vi "DriveForDistanceController.vi"(0 "Distance":dbl=300.0, 5 "Angle":dbl=164.32, 9 "SensorData":T3={"LeftDistance"=261.910213470459, "RightDistance"=383.47772216796875, "LeftVelocity"=63.071308056640625, "RightVelocity"=41.74135772460938, "Angle"=164.32, "Location"={-465.44436408260333, -5.658206958861253}}, 11 "Gains":T2={"FFV"=0.0097, "FFA"=0.002, "Vel PID"={"P"=0.0, "I"=0.0, "D"=0.0}}, 12 "Trackwidth":dbl=25.0 format="%#_13g", 13 "Reset":bool) -> (4 "Left Speed":dbl, 6 "Right Speed":dbl=-2.7755575615628914e-17, 10 "Done":bool=TRUE, 14 "Graph":cluster{cluster{"x":dbl, "y":dbl}[]}[](graph)=[{[{"x"=-182.84036380917772, "y"=-102.60157058324037}, {"x"=-188.50213040089133, "y"=-100.61551946079776}, {"x"=-194.16389699260495, "y"=-98.62946833835514}, {"x"=-199.82566358431856, "y"=-96.64341721591252}, {"x"=-205.48743017603218, "y"=-94.65736609346989}, {"x"=-211.1491967677458, "y"=-92.67131497102727}, {"x"=-216.8109633594594, "y"=-90.68526384858465}, {"x"=-222.47272995117302, "y"=-88.69921272614204}, {"x"=-228.13449654288664, "y"=-86.71316160369942}, {"x"=-233.79626313460025, "y"=-84.7271104812568}, {"x"=-239.45802972631387, "y"=-82.74105935881417}, {"x"=-245.11979631802748, "y"=-80.75500823637157}, {"x"=-250.7815629097411, "y"=-78.76895711392893}, {"x"=-256.44332950145474, "y"=-76.78290599148632}, {"x"=-262.1050960931683, "y"=-74.7968548690437}, {"x"=-267.76686268488197, "y"=-72.81080374660108}, {"x"=-273.42862927659553, "y"=-70.82475262415846}, {"x"=-279.0903958683092, "y"=-68.83870150171583}, {"x"=-284.75216246002276, "y"=-66.85265037927323}, {"x"=-290.41392905173643, "y"=-64.8665992568306}, {"x"=-296.07569564345, "y"=-62.88054813438798}, {"x"=-301.73746223516366, "y"=-60.89449701194536}, {"x"=-307.3992288268772, "y"=-58.908445889502744}, {"x"=-313.0609954185909, "y"=-56.922394767060126}, {"x"=-318.72276201030445, "y"=-54.9363436446175}, {"x"=-324.3845286020181, "y"=-52.950292522174884}, {"x"=-330.0462951937317, "y"=-50.964241399732266}, {"x"=-335.70806178544535, "y"=-48.97819027728964}, {"x"=-341.3698283771589, "y"=-46.992139154847024}, {"x"=-347.0315949688726, "y"=-45.006088032404406}, {"x"=-352.69336156058614, "y"=-43.02003690996179}, {"x"=-358.3551281522998, "y"=-41.033985787519164}, {"x"=-364.01689474401337, "y"=-39.047934665076546}, {"x"=-369.67866133572704, "y"=-37.06188354263392}, {"x"=-375.3404279274406, "y"=-35.075832420191304}, {"x"=-381.0021945191543, "y"=-33.08978129774869}, {"x"=-386.66396111086783, "y"=-31.10373017530607}, {"x"=-392.3257277025815, "y"=-29.11767905286345}, {"x"=-397.98749429429506, "y"=-27.131627930420834}, {"x"=-403.64926088600873, "y"=-25.145576807978216}, {"x"=-409.3110274777223, "y"=-23.159525685535584}, {"x"=-414.97279406943596, "y"=-21.173474563092967}, {"x"=-420.6345606611495, "y"=-19.18742344065035}, {"x"=-426.2963272528632, "y"=-17.20137231820773}, {"x"=-431.95809384457675, "y"=-15.215321195765114}, {"x"=-437.6198604362904, "y"=-13.229270073322496}, {"x"=-443.281627028004, "y"=-11.243218950879879}, {"x"=-448.94339361971765, "y"=-9.257167828437247}, {"x"=-454.6051602114312, "y"=-7.271116705994629}, {"x"=-460.2669268031449, "y"=-5.2850655835520115}, {"x"=-461.21055456843044, "y"=-4.954057063144916}, {"x"=-465.92869339485844, "y"=-3.299014461109394}]}, {[{"x"=-465.44436408260333, "y"=-5.658206958861253}, {"x"=-476.9977978243892, "y"=-2.415034318657715}]}, {[{"x"=-463.7557202118273, "y"=-4.061256379649985}]}, {[{"x"=-440.44436408260333, "y"=-5.658206958861253}, {"x"=-440.9906740642582, "y"=-0.46041468841727085}, {"x"=-442.6057276415383, "y"=4.51020911803375}, {"x"=-445.21893922322965, "y"=9.036424348450575}, {"x"=-448.7160989236319, "y"=12.9204136780736}, {"x"=-452.94436408260333, "y"=15.992428135749712}, {"x"=-457.71893922322965, "y"=18.118205948517584}, {"x"=-462.83115250091197, "y"=19.20484042534558}, {"x"=-468.0575756642947, "y"=19.20484042534558}, {"x"=-473.169788941977, "y"=18.118205948517588}, {"x"=-477.94436408260333, "y"=15.992428135749716}, {"x"=-482.1726292415748, "y"=12.920413678073608}, {"x"=-485.669788941977, "y"=9.036424348450577}, {"x"=-488.28300052366836, "y"=4.510209118033757}, {"x"=-489.89805410094846, "y"=-0.4604146884172602}, {"x"=-490.44436408260333, "y"=-5.658206958861251}, {"x"=-489.89805410094846, "y"=-10.85599922930523}, {"x"=-488.28300052366836, "y"=-15.82662303575625}, {"x"=-485.669788941977, "y"=-20.35283826617308}, {"x"=-482.1726292415748, "y"=-24.236827595796104}, {"x"=-477.94436408260333, "y"=-27.308842053472212}, {"x"=-473.169788941977, "y"=-29.43461986624009}, {"x"=-468.0575756642947, "y"=-30.521254343068087}, {"x"=-462.831152500912, "y"=-30.521254343068087}, {"x"=-457.71893922322965, "y"=-29.434619866240094}, {"x"=-452.94436408260333, "y"=-27.30884205347223}, {"x"=-448.7160989236319, "y"=-24.236827595796118}, {"x"=-445.21893922322965, "y"=-20.352838266173087}, {"x"=-442.6057276415383, "y"=-15.826623035756276}, {"x"=-440.9906740642582, "y"=-10.855999229305251}, {"x"=-440.44436408260333, "y"=-5.65820695886126}]}, {[{"x"=-266.3585601807637, "y"=145.23719379541097}, {"x"=-269.7834396945887, "y"=177.82274570174297}, {"x"=-279.90839456691435, "y"=208.98415262694203}, {"x"=-296.29091568489616, "y"=237.35951155935658}, {"x"=-318.21500826362, "y"=261.70868315356114}, {"x"=-344.72248425392746, "y"=280.96749177060053}, {"x"=-374.65483975805995, "y"=294.29423505989314}, {"x"=-406.7038872091095, "y"=301.10647039088764}, {"x"=-439.46892944507306, "y"=301.1064703908877}, {"x"=-471.5179768961226, "y"=294.2942350598932}, {"x"=-501.4503324002551, "y"=280.96749177060053}, {"x"=-527.9578083905625, "y"=261.7086831535612}, {"x"=-549.8819009692864, "y"=237.35951155935658}, {"x"=-566.2644220872683, "y"=208.9841526269421}, {"x"=-576.3893769595938, "y"=177.82274570174303}, {"x"=-579.8142564734189, "y"=145.237193795411}, {"x"=-576.3893769595938, "y"=112.651641889079}, {"x"=-566.2644220872683, "y"=81.49023496387996}, {"x"=-549.8819009692864, "y"=53.114876031465386}, {"x"=-527.9578083905626, "y"=28.76570443726081}, {"x"=-501.4503324002552, "y"=9.506895820221445}, {"x"=-471.51797689612266, "y"=-3.8198474690712203}, {"x"=-439.46892944507323, "y"=-10.632082800065689}, {"x"=-406.7038872091096, "y"=-10.632082800065717}, {"x"=-374.65483975806, "y"=-3.8198474690712487}, {"x"=-344.7224842539276, "y"=9.506895820221331}, {"x"=-318.2150082636201, "y"=28.765704437260723}, {"x"=-296.29091568489616, "y"=53.11487603146533}, {"x"=-279.90839456691447, "y"=81.49023496387979}, {"x"=-269.7834396945887, "y"=112.65164188907889}, {"x"=-266.3585601807637, "y"=145.23719379541095}]}], 15 "Time Left":dbl=20.0)   [LabVIEW 2020]
uses:
  PurePursuit/RobotNeededPathData.ctl
panel:
  out "outputs":T1(graph)={"LeftValue"=0.0, "RightValue"=-2.7755575615628914e-17, 1.0, 0.5}
  out "Vel vs Target Vel":cluster{dbl, "TargetVel":dbl}(graph)={52.406332890625, "TargetVel"=52.70905958272918}
  in  "MaxDeAccel":dbl=120.0 format="%#_13g"
  in  "LookaheadDist":dbl=25.0
  in  "SlowSpeed":dbl=30.0 format="%#_13g"
  in  "SlowDistanceAtEnd":dbl=12.0 format="%#_13g"
  in  "MaxAccel":dbl=120.0
  in  "MaxVel":dbl=70.0
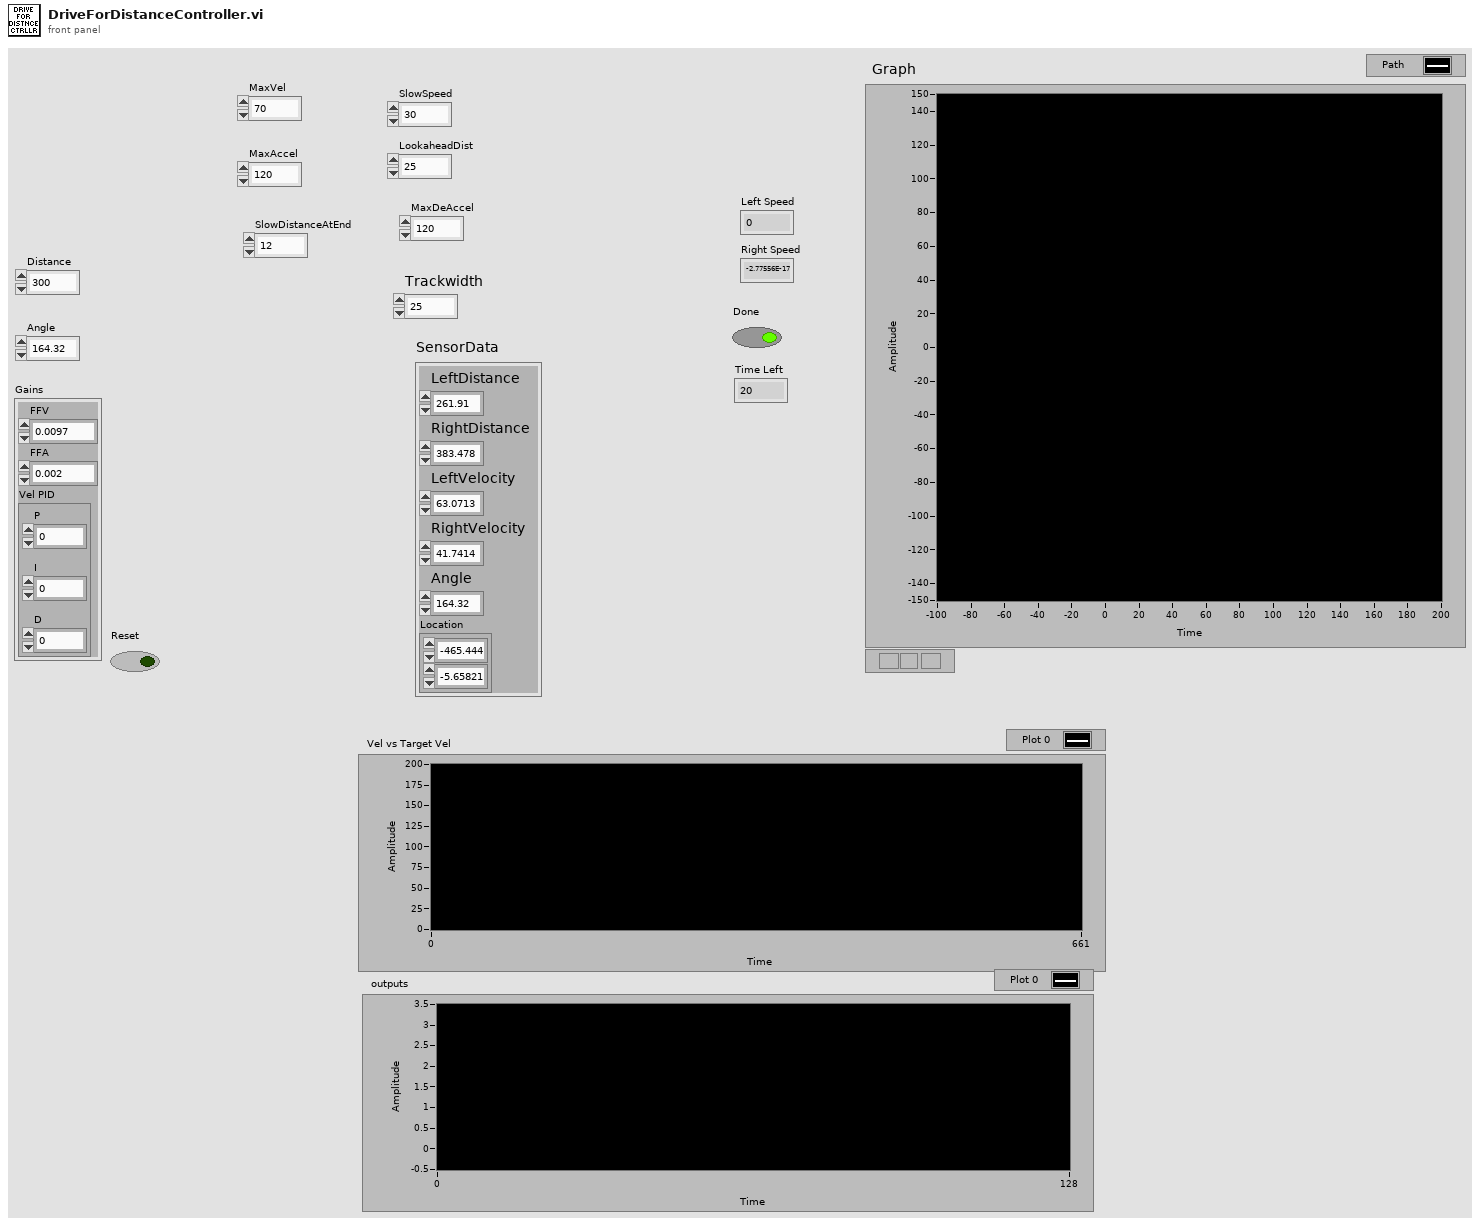
[diagram p1: front panel]
types:
  T1 = cluster{"LeftValue":dbl, "RightValue":dbl, dbl, dbl}
  T2 = cluster{"FFV":dbl, "FFA":dbl, "Vel PID":cluster{"P":dbl, "I":dbl, "D":dbl}}
  T3 = cluster{"LeftDistance":dbl, "RightDistance":dbl, "LeftVelocity":dbl, "RightVelocity":dbl, "Angle":dbl, "Location":cluster{dbl, dbl}}
  T4 = typedef "RobotNeededPathData.ctl" = cluster{"Path":cluster{dbl, dbl}[], "MaxVel":dbl, "MaxAccel":dbl, "Backwards?":bool, "PointSpacing":dbl, "LookaheadDist":dbl, "Speed/Curve":dbl, "SlowDistanceAtEnd":dbl, "SlowSpeed":dbl, "MaxDeAccel":dbl}
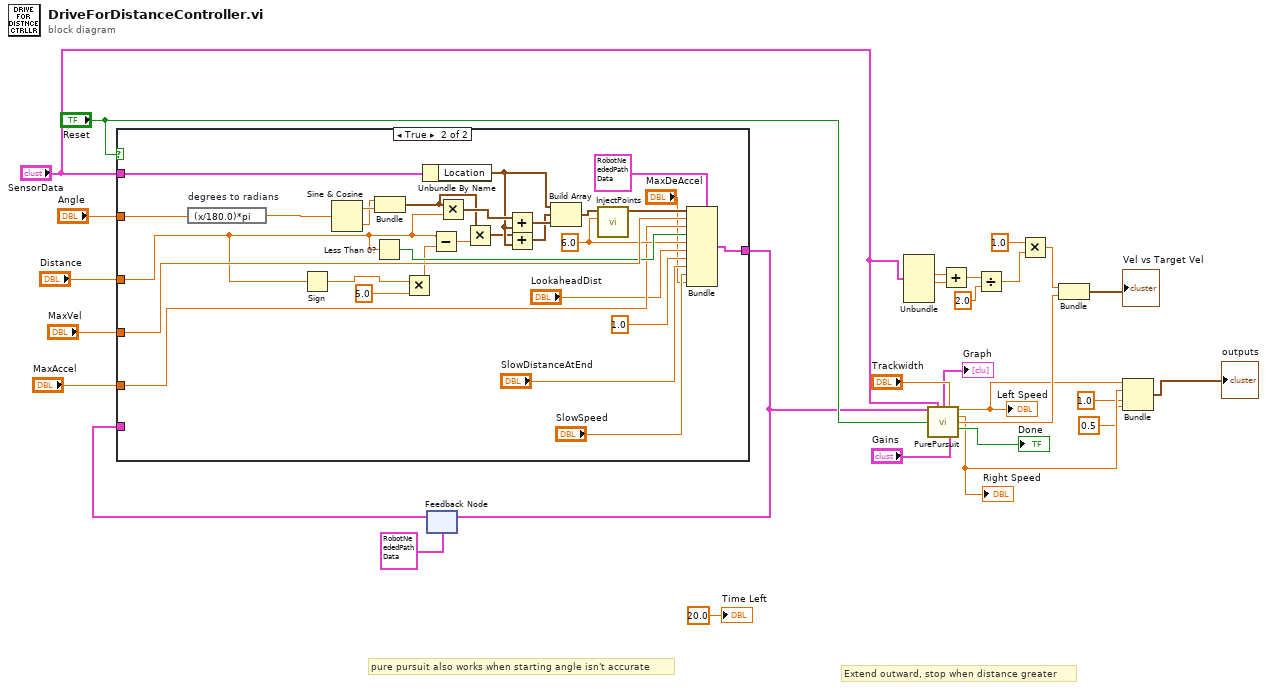
[diagram p0: block diagram]
diagram:
  # "pure pursuit also works when starting angle isn't accurate"
  # "Extend outward, stop when distance greater"
  n1 = feedback #1(T4 {"Path"=[], "MaxVel"=0.0, "MaxAccel"=0.0, "Backwards?"=FALSE, "PointSpacing"=0.0, "LookaheadDist"=0.0, "Speed/Curve"=1.8, "SlowDistanceAtEnd"=12.0, "SlowSpeed"=15.0, "MaxDeAccel"=0.0} ("RobotNeededPathData")) -> (w23:T4)
  n2 = case shown="True" "Reset" {
    tunnel: "SensorData" -> [_ w58]
    tunnel: "Angle" -> [_ w30]
    tunnel: "Distance" -> [_ w34]
    tunnel: "MaxVel" -> [_ w50]
    tunnel: "MaxAccel" -> [_ w46]
    tunnel: [w29 w42] -> w21
    tunnel: w23 -> [w29 _]
    frame False {
    }
    frame True {
      w48 = 6.0 ("Spacing")
      n3 = expression code="(x/180.0)*pi" "degrees to radians"(w30) -> (w57:dbl)
      n4 = Sign(1:w34) -> (0:w35:dbl)
      n5 = Sine & Cosine(0:w57) -> (1:w56:dbl, 2:w55:dbl)
      n6 = Less Than 0?(x=w34) -> (x < 0?=w49:bool)
      n7 = Bundle(w55, w56) -> (w41:cluster{dbl, dbl})  [unwired: 1 in]
      n8 = Multiply(x=w35, y=5.0) -> (x*y=w33:dbl)
      n9 = Unbundle By Name(w58) -> ("Location"=w40:cluster{dbl, dbl})
      n10 = Subtract(x=w34, y=w33) -> (x-y=w38:dbl)
      n11 = Multiply(x=w41, y=w34) -> (x*y=w54:cluster{dbl, dbl})
      n12 = Multiply(x=w41, y=w38) -> (x*y=w39:cluster{dbl, dbl})
      n13 = Add(x=w54, y=w40) -> (x+y=w32:cluster{dbl, dbl})
      n14 = Add(x=w39, y=w40) -> (x+y=w31:cluster{dbl, dbl})
      n15 = Build Array(w40, w31, w32) -> (w53:cluster{dbl, dbl}[])
      n16 = call "InjectPoints.vi"("Spacing"=w48, "Path"=w53) -> ("Path out"=w51:cluster{dbl, dbl}[])  [unwired: 9 in]
      n17 = Bundle(cluster=T4 {"Path"=[], "MaxVel"=0.0, "MaxAccel"=0.0, "Backwards?"=FALSE, "PointSpacing"=0.0, "LookaheadDist"=0.0, "Speed/Curve"=1.8, "SlowDistanceAtEnd"=12.0, "SlowSpeed"=15.0, "MaxDeAccel"=0.0} ("RobotNeededPathData"), "Path"=w51, "MaxVel"=w50, "MaxAccel"=w46, "Backwards?"=w49, "PointSpacing"=w48, "LookaheadDist"="LookaheadDist", "Speed/Curve"=1.0, "SlowDistanceAtEnd"="SlowDistanceAtEnd", "SlowSpeed"="SlowSpeed", "MaxDeAccel"="MaxDeAccel") -> (w42:T4)
    }
  }
  n18 = feedback-in #1(w21) -> ()
  n19 = Unbundle("SensorData") -> ("LeftVelocity"=w13:dbl, "RightVelocity"=w14:dbl)  [unwired: 4 out]
  n20 = call "PurePursuit.vi"("RobotNeededPathData"=w21, "SensorData"="SensorData", "Trackwidth"="Trackwidth", "Reset"="Reset", "Gains"="Gains") -> ("Graph"=→"Graph":cluster{cluster{"x":dbl, "y":dbl}[]}[], "LeftValue"=w5:dbl, "RightValue"=w4:dbl, "TargetVel"=w10:dbl, "Done"=→"Done":bool)  [unwired: 6 in]
  "Left Speed" <- w5
  "Right Speed" <- w4
  n21 = Add(x=w13, y=w14) -> (x+y=w12:dbl)
  n22 = Divide(x=w12, y=2.0) -> (x/y=w6:dbl)
  n23 = Multiply(x=1.0, y=w6) -> (x*y=w8:dbl)
  n24 = Bundle(w8, "TargetVel"=w10) -> (→"Vel vs Target Vel":cluster{dbl, "TargetVel":dbl})  [unwired: 1 in]
  n25 = Bundle("LeftValue"=w5, "RightValue"=w4, 1.0, 0.5) -> (→"outputs":T1)  [unwired: 1 in]
  "Time Left" <- 20.0 ("Time Left")
